vi "niDTS WLAN DSSS Tx Test Set Parameters.vi"(0 "Dummy Test Handle in":T12, 7 "Parameters":T1={"DSSS Data Rate (Mbps)"=enum."11", "Chains"=[TRUE, FALSE, FALSE, FALSE], "Bandwidth (Hz)"=enum."20 MHz", "Channel"=1, "Dut Tx Power  (dBm)"=0.0, "16 symbols"=TRUE, "Payload Length (bytes)"=1, "Idle Interval (s)"=0.0, "External Attenuation (dB)"=[0.0, 0.0, 0.0, 0.0], "Acquisition "={"Acquisition Length Mode"=enum."AUTO", "Acquisition Length (s)"=3.0, "Auto Level"=FALSE}, "TXP Measurement"={"TXP Power Enable"=FALSE, "TXP Averages"=3}, "ModAcc Measurement"={"ModAcc Enable"=FALSE, "Header Detection"=enum."FIRST", "Averages"=3, "CFO Estimation"=enum."PAMBLE", "DC Offset Compensation"=FALSE, "Chip Start Location"=0, "Max Chips Used"=16, "Pulse Shaping FilterType"=enum."GAUSSIAN", "Pulse Shaping Filter Coefficient"=0.35, "Equalization"=TRUE, "Phase Tracking"=TRUE}, "SEM Measurement"={"SEM Enable"=FALSE, "SEM Averages"=3, "Auto Span Enable"=FALSE, "Frequency Span (Hz)"=0.0, "Measurement Type"=enum."Standard", "Mask Frequencies (Hz)"=[], "Mask Power Offsets (dB)"=[]}, "OBW Measurement"={"OBW Enable"=FALSE, "OBW Averages"=3}, "DSSS Power Ramp"={"Power Ramp Enable"=FALSE, "Averages"=3, "Thresholds"={"Up Low (%)"=10.0, "Down Low (%)"=10.0, "Up High (%)"=90.0, "Down High (%)"=90.0}}} {"DSSS Power Ramp"."Thresholds"."Down High (%)" min=0.0 max=100.0 step=1.0; "DSSS Power Ramp"."Thresholds"."Up High (%)" min=0.0 max=100.0 step=1.0; "DSSS Power Ramp"."Thresholds"."Down Low (%)" min=0.0 max=100.0 step=1.0; "DSSS Power Ramp"."Thresholds"."Up Low (%)" min=0.0 max=100.0 step=1.0; "Acquisition"."Acquisition Length (s)" format="%#_6p"; "SEM Measurement"."Frequency Span (Hz)" format="%#_6p"; "Channel" items=["1"=1, "2"=2, "3"=3, "4"=4, "5"=5, "6"=6, "7"=7, "8"=8, "9"=9, "10"=10, "11"=11, "12"=12, "13"=13, "14"=14]; "Idle Interval (s)" format="%_3p"}, 11 "error in (no error)":errorcluster) -> (4 "Dummy Test Handle out":T12, 15 "error out":errorcluster)   [LabVIEW 2014, in "niDTS WLAN.lvlib"]
uses:
  niDTS WLAN.lvlib
  Tx Test/Includes/niDTS WLAN Tx Test INC Handle.ctl
  Tx Test/Objects/BASE_class/niDTS WLAN Tx Test.lvclass
  Includes/niDTS WLAN DSSS Tx Test INC Parameters.ctl
  Includes/niDTS WLAN INC DSSS Data Rate.ctl
  Includes/niDTS WLAN INC CH BW DSSS.ctl
  Includes/niDTS WLAN INC Channel DSSS.ctl
  Includes/niDTS WLAN DUT INC Acquisition Parameters.ctl
  Includes/niDTS WLAN INC TXP Measurement Parameters.ctl
  Includes/niDTS WLAN DSSS Tx Test INC ModAcc Measurement Parameters.ctl
  Includes/niDTS WLAN INC Pulse Shaping Filter Type.ctl
  Includes/niDTS WLAN INC SEM Measurement Parameters.ctl
  Includes/niDTS WLAN INC OBW Measurement Parameters.ctl
  Includes/niDTS WLAN INC DSSS Power Ramp Parameters.ctl
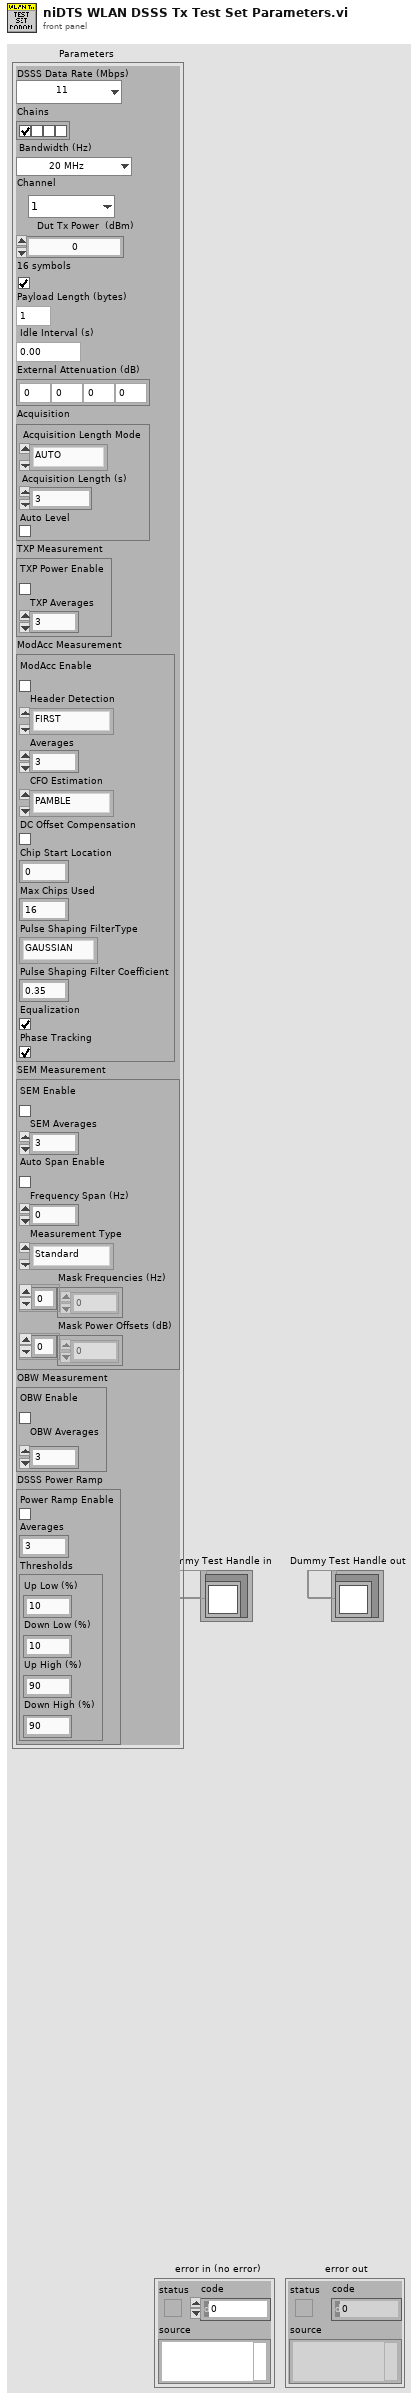
[diagram p1: front panel]
types:
  T1 = typedef "niDTS WLAN.lvlib/niDTS WLAN DSSS Tx Test INC Parameters.ctl" = cluster{"DSSS Data Rate (Mbps)":T2, "Chains":bool[], "Bandwidth (Hz)":T3, "Channel":T4, "Dut Tx Power  (dBm)":dbl, "16 symbols":bool, "Payload Length (bytes)":i32, "Idle Interval (s)":dbl, "External Attenuation (dB)":dbl[], "Acquisition ":T5, "TXP Measurement":T6, "ModAcc Measurement":T7, "SEM Measurement":T9, "OBW Measurement":T10, "DSSS Power Ramp":T11}
  T2 = typedef "niDTS WLAN.lvlib/niDTS WLAN INC DSSS Data Rate.ctl" = enum16{"1", "2", "5.5", "11"}
  T3 = typedef "niDTS WLAN.lvlib/niDTS WLAN INC CH BW DSSS.ctl" = enum16{"20 MHz"}
  T4 = typedef "niDTS WLAN.lvlib/niDTS WLAN INC Channel DSSS.ctl" = i8
  T5 = typedef "niDTS WLAN.lvlib/niDTS WLAN DUT INC Acquisition Parameters.ctl" = cluster{"Acquisition Length Mode":enum16{"AUTO", "MANUAL"}, "Acquisition Length (s)":dbl, "Auto Level":bool}
  T6 = typedef "niDTS WLAN.lvlib/niDTS WLAN INC TXP Measurement Parameters.ctl" = cluster{"TXP Power Enable":bool, "TXP Averages":i32}
  T7 = typedef "niDTS WLAN.lvlib/niDTS WLAN DSSS Tx Test INC ModAcc Measurement Parameters.ctl" = cluster{"ModAcc Enable":bool, "Header Detection":enum16{"MANUAL", "FIRST", "ALL"}, "Averages":i32, "CFO Estimation":enum16{"PAMBLE", "PDATA"}, "DC Offset Compensation":bool, "Chip Start Location":i16, "Max Chips Used":i16, "Pulse Shaping FilterType":T8, "Pulse Shaping Filter Coefficient":dbl, "Equalization":bool, "Phase Tracking":bool}
  T8 = typedef "niDTS WLAN.lvlib/niDTS WLAN INC Pulse Shaping Filter Type.ctl" = enum16{"NONE", "RCOSINE", "RRCOSINE", "GAUSSIAN"}
  T9 = typedef "niDTS WLAN.lvlib/niDTS WLAN INC SEM Measurement Parameters.ctl" = cluster{"SEM Enable":bool, "SEM Averages":i32, "Auto Span Enable":bool, "Frequency Span (Hz)":dbl, "Measurement Type":enum16{"Standard", "Legacy", "Custom"}, "Mask Frequencies (Hz)":dbl[], "Mask Power Offsets (dB)":dbl[]}
  T10 = typedef "niDTS WLAN.lvlib/niDTS WLAN INC OBW Measurement Parameters.ctl" = cluster{"OBW Enable":bool, "OBW Averages":i32}
  T11 = typedef "niDTS WLAN.lvlib/niDTS WLAN INC DSSS Power Ramp Parameters.ctl" = cluster{"Power Ramp Enable":bool, "Averages":i32, "Thresholds":cluster{"Up Low (%)":dbl, "Down Low (%)":dbl, "Up High (%)":dbl, "Down High (%)":dbl}}
  T12 = typedef "niDTS WLAN.lvlib/niDTS WLAN Tx Test INC Handle.ctl" = refnum<data-value>
  T13 = typedef "niDTS WLAN.lvlib/niDTS WLAN Tx Test INC Parameters.ctl" = cluster{"Standard":T14, "DSSS Data Rate (Mbps)":T2, "OFDM Data Rate (Mbps)":T15, "MCS Index":i32, "N spatial streams":i32, "Chains":bool[], "BandWidth (Hz)":T16, "Channel":i32, "Gard Interval":T17, "FEC Coding":T18, "Dut Tx Power":dbl, "16 symbols":bool, "payload length bytes":i32, "idle interval":dbl, "External Attenuation":dbl[], "Acquisition Parameters ":T5, "TXP Measurement Parameters":T6, "ModAcc Measurement Paramaters":T19, "ModAcc DSSS Paramaters":T20, "SEM Measurement Parameters":T9, "OBW Measurement Parameters":T10, "DSSS Power Ramp":T11, "Enable Traces":bool}
  T14 = typedef "niDTS WLAN.lvlib/niDTS WLAN INC Standard.ctl" = enum16{"802.11 b DSSS", "802.11 a/g OFDM", "802.11 n HT", "802.11 ac VHT"}
  T15 = typedef "niDTS WLAN.lvlib/niDTS WLAN INC OFDM Data Rate.ctl" = enum16{"6", "9", "12", "18", "24", "36", "48", "54"}
  T16 = typedef "niDTS WLAN.lvlib/niDTS WLAN INC CH BW.ctl" = enum16{"20 MHz", "40 MHz", "80 MHz", "160 MHz"}
  T17 = typedef "niDTS WLAN.lvlib/niDTS WLAN INC GI.ctl" = enum16{"LONG", "SHORT"}
  T18 = typedef "niDTS WLAN.lvlib/niDTS WLAN INC FEC Coding.ctl" = enum16{"BCC", "LDPC"}
  T19 = typedef "niDTS WLAN.lvlib/niDTS WLAN INC ModAcc Measurement Parameters.ctl" = cluster{"ModAcc Enable":bool, "Header Detection":enum16{"MANUAL", "FIRST", "ALL"}, "Averages":i32, "Amplitude Tracking":bool, "Channel Tracking":bool, "Time Tracking":bool, "Phase Tracking":enum16{"NONE", "STANDARD", "CSF", "INSTANT"}, "Clock Offset Est":bool, "Impairments Est":bool, "CFO Estimation":enum16{"PAMBLE", "PDATA"}}
  T20 = typedef "niDTS WLAN.lvlib/niDTS WLAN INC DSSS ModAcc Measurement Parameters.ctl" = cluster{"DC Offset Compensation":bool, "Equalization":bool, "Phase Tracking":bool, "Chip Start Location":i16, "Max Chips Used":i16, "Pulse Shaping FilterType":T8, "Pulse Shaping Filter Coefficient":dbl}
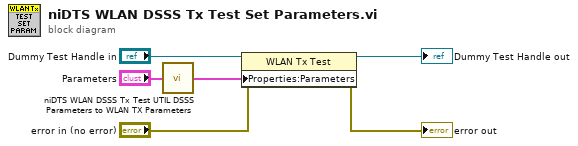
[diagram p0: block diagram]
diagram:
  n1 = call "niDTS WLAN DSSS Tx Test UTIL DSSS Parameters to WLAN TX Parameters.vi"("DSSS Parameters"="Parameters") -> ("WLAN Tx Parameters"=w2:T13)  [unwired: 14 in]
  n2 = property class="WLAN Tx Test"(reference="Dummy Test Handle in", error in="error in (no error)", "Properties:Parameters"=w2) -> (reference out=→"Dummy Test Handle out":T12, error out=→"error out":errorcluster)
